vi "TestRelays.vi"() -> (0 "Error Out":errorcluster)   [LabVIEW 2018]
panel:
  in  "Sample Space Pump":bool
  in  "Siphon Pump":bool
  in  "Neutron Shutter":bool
  in  "stop":bool
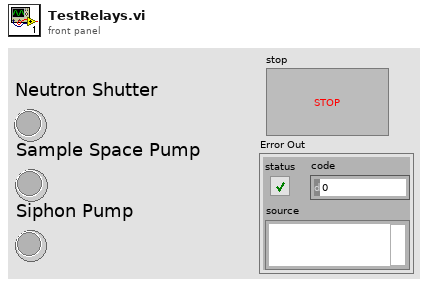
[diagram p1: front panel]
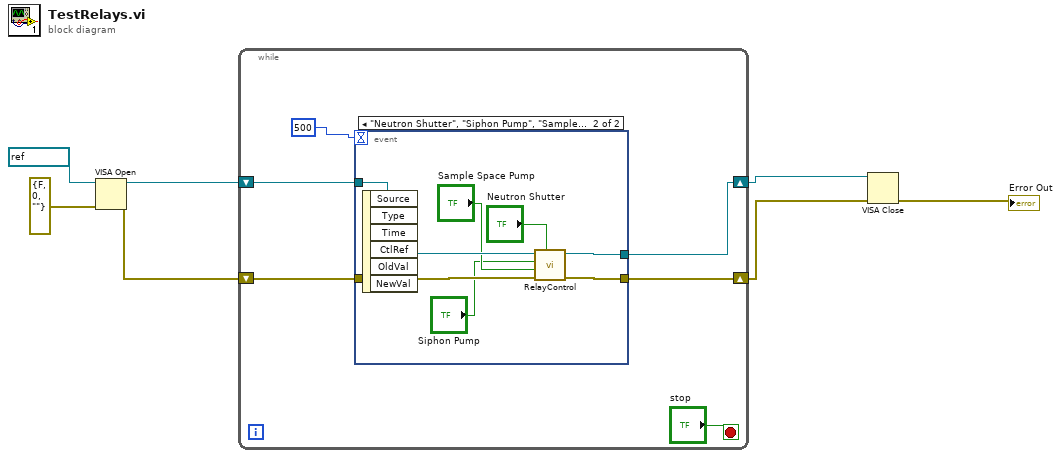
[diagram p0: block diagram]
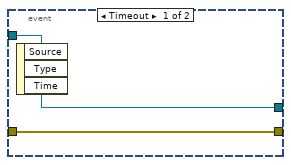
[diagram p2: hidden frame]
diagram:
  n1 = VISA Open(error in (no error)=errorcluster {"status"=FALSE, "code"=0, "source"=""}, VISA resource name=refnum<visa-resource-name> "Relays") -> (VISA resource name=w4:refnum<visa-resource-name>, error out=w3:errorcluster)  [unwired: 3 in]
  n2 = while {
    shift-right: [w10] -> w2
    shift-left: w4 -> [w12]
    shift-right: [w9] -> w1
    shift-left: w3 -> [w11]
    stop <- "stop" stop-if-true
    n3 = event shown="[1] \"Neutron Shutter\", \"Siphon Pump\", \"Sample Space Pump\": Value Change" {
      selector: _ -> [_ _]
      dyn-events: _ -> [_ _]
      timeout: u32 500 ("milliseconds to wait") -> [_ _]
      tunnel: w12 -> [w14 w22]
      tunnel: w11 -> [w15 w21]
      tunnel: [w14 w20] -> w10
      tunnel: [w15 w19] -> w9
      event Timeout {
        n4 = event-data() -> ()  [unwired: 1 in, 3 out]
      }
      event "Neutron Shutter", "Siphon Pump", "Sample Space Pump": Value Change {
        n5 = event-data() -> ()  [unwired: 1 in, 6 out]
        n6 = call "RelayControl.vi"("Neutron Shutter"="Neutron Shutter", "Error In"=w21, "Sample Space Pump"="Sample Space Pump", "Siphon Pump"="Siphon Pump", "Relay In"=w22) -> ("Error Out"=w19:errorcluster, "Relay Out"=w20:refnum<visa-resource-name>)  [unwired: 5 in]
      }
    }
  }
  n7 = VISA Close(VISA resource name=w2, error in (no error)=w1) -> (error out=→"Error Out":errorcluster)
